vi "Filter Only Eulogy.vi"(8 "Error In":errorcluster, 11 "VI Bookmarks":T1[](array[typedef])) -> (0 "Error Out":errorcluster, 3 "Eulogy Bookmarks":T1[](array[typedef]))   [LabVIEW 2017, in "Graveyard.lvlib"]
doc: "Filters out all bookmarks that are NOT graves"
uses:
  Graveyard.lvlib
  VI Bookmark.ctl
  VI Information.ctl
  Application Information.ctl
  Eulogy/Public/Bookmarks.ctl
  Eulogy/Eulogy.lvlib
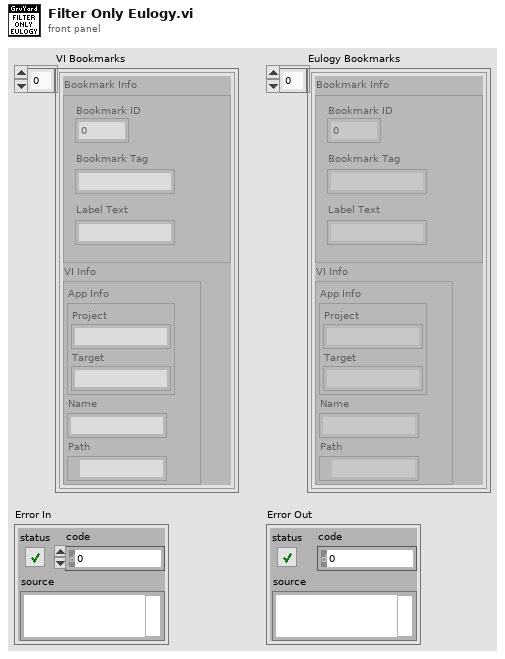
[diagram p1: front panel]
types:
  T1 = typedef "Graveyard.lvlib/VI Bookmark.ctl" = cluster{"Bookmark Info":cluster{"Bookmark ID":u32, "Bookmark Tag":string, "Label Text":string}, "VI Info":T2}
  T2 = typedef "Graveyard.lvlib/VI Information.ctl" = cluster{"App Info":T3, "Name":string, "Path":path}
  T3 = typedef "Graveyard.lvlib/Application Information.ctl" = cluster{"Project":string, "Target":string}
  T4 = typedef "Eulogy.lvlib/Bookmarks.ctl" = enum16{"RIP", "Zombie"}
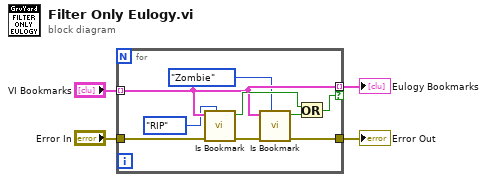
[diagram p0: block diagram]
diagram:
  n1 = for {
    tunnel: "VI Bookmarks" -> [w10] mode=indexing
    tunnel: [w10] -> w1 mode=indexing if=w13
    tunnel: "Error In" -> [w9]
    tunnel: [w7] -> w3
    n2 = call "Is Bookmark.vi"("Bookmark"=Bookmarks."RIP", "Error In"=w9, "VI Bookmark"=w10) -> ("Error Out"=w8:errorcluster, "Is Bookmark"=w11:bool)  [unwired: 7 in]
    n3 = call "Is Bookmark.vi"("Bookmark"=Bookmarks."Zombie", "Error In"=w8, "VI Bookmark"=w10) -> ("Error Out"=w7:errorcluster, "Is Bookmark"=w12:bool)  [unwired: 7 in]
    n4 = Or(x=w11, y=w12) -> (x .or. y?=w13:bool)
  }
  "Error Out" <- w3
  "Eulogy Bookmarks" <- w1
